vi "Custom Selection.vi"(4 "error in (no error)":errorcluster caption="错误输入（无错误）", 5 "Value":bool[](array[boolean]), 6 "Container State":T1 caption="容器状态", 7 "Display State In":T2 caption="显示状态输入") -> (0 "error out":errorcluster caption="错误输出", 3 "Display State Out":T2 caption="显示状态输出")   [LabVIEW 2018, in "ListBox XControl.xctl"]
uses:
  ListBox XControl.xctl
  <vilib>/_xctls/Container State.ctl
  State ListBox.ctl
  <vilib>/_xctls/XControlSupport.lvlib
panel:
  in  "Container State 2":T1
  # "将以下值显示控件替换为所需类型的显示控件。\n不要从连线板中删除该显示控件或其它显示控件。\n不要更改连线板模式。\n值显示控件应始终位于连线板输出端自顶部起第三个接线端。"
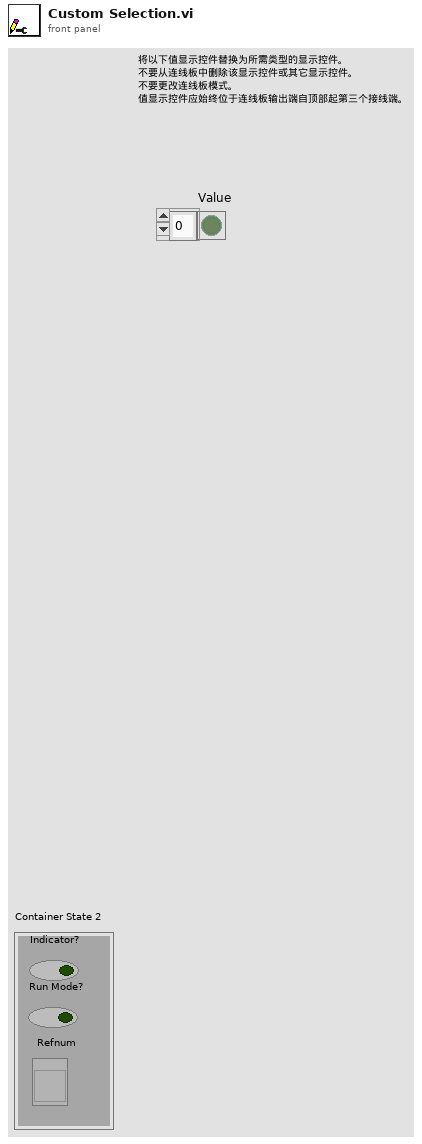
[diagram p1: front panel]
types:
  T1 = typedef "XControlSupport.lvlib/Container State.ctl" = cluster{"Indicator?":bool, "Run Mode?":bool, " Refnum":refnum<vi>}
  T2 = typedef "ListBox XControl.xctl/State ListBox.ctl" = cluster{"ItemNames[]":string[], "Listbox Ref":refnum<vi>, "Select All By Default":bool}
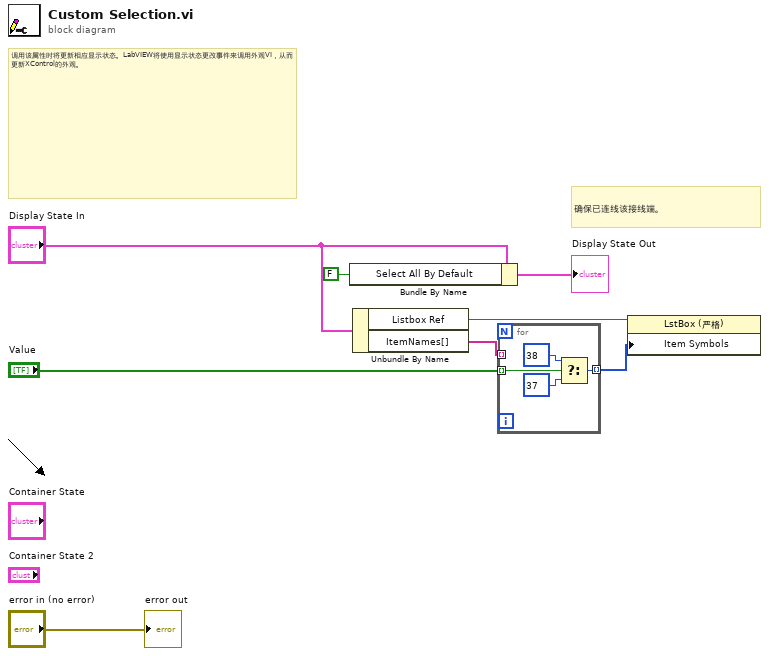
[diagram p0: block diagram]
diagram:
  # "确保已连线该接线端。"
  # "调用该属性时将更新相应显示状态。LabVIEW将使用显示状态更改事件来调用外观VI，从而更新XControl的外观。"
  n1 = Bundle By Name(cluster="Display State In", "Select All By Default"=FALSE) -> (→"Display State Out":T2)
  n2 = Unbundle By Name("Display State In") -> ("Listbox Ref"=w7:refnum<vi>, "ItemNames[]"=w6:string[])
  n3 = for {
    tunnel: w6 -> [_] mode=indexing
    tunnel: [w10] -> w5 mode=indexing
    tunnel: "Value" -> [w9] mode=indexing
    n4 = Select(t=38, s=w9, f=37) -> (s? t:f=w10:i32)
  }
  n5 = property class="LstBox (严格)"(reference=w7, "Item Symbols"=w5) -> ()  [unwired: 1 in, 2 out]
  "error out" <- "error in (no error)"
